vi "DAQmx_AnalogInput_MultiChannel.vi"() -> ()   [LabVIEW 2025]
panel:
  in  "stop":bool
  out "data":dynamicdata(graph)
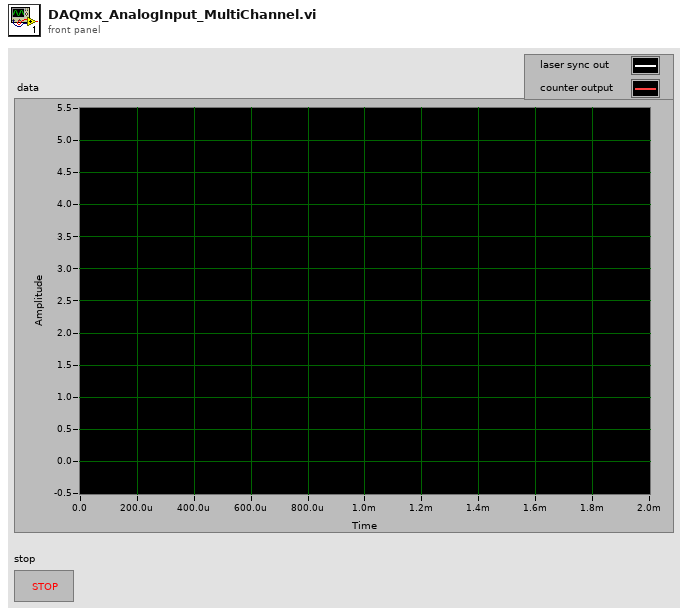
[diagram p1: front panel]
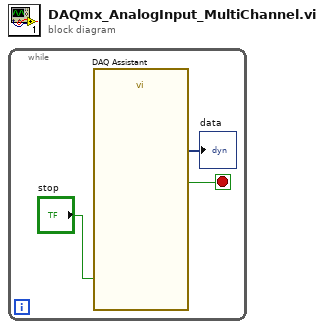
[diagram p0: block diagram]
diagram:
  n1 = while {
    stop <- w3 stop-if-true
    n2 = call "DAQ Assistant"("stop (F)"="stop") -> ("data"=→"data":dynamicdata, "stopped"=w3:bool)  [unwired: 15 in, 2 out]
  }
